vi "NF87XX.ProcCases.vi"(0 "i ref in":refnum<vi>, 1 "selector":string, 2 "Data":T1, 3 "call cluster":T2={"Object"="", "Selector"="", "CallType"=enum."synchronous", "Async Object"="", "Async Selector"="", "Data Descriptor"="", "Data"=[], "Error #"=0, "Expire"=0}, 5 "error in":errorcluster) -> (14 "i ref out":refnum<vi>, 17 "answer cluster":T2={"Object"="", "Selector"="", "CallType"=enum."synchronous", "Async Object"="", "Async Selector"="", "Data Descriptor"="", "Data"=[], "Error #"=0, "Expire"=0}, 19 "error out":errorcluster)   [LabVIEW 2014, in "NF87XX.lvlib"]
doc: "This method is called by a process from within the default case in the event loop. The methods of a class that are linked to events will be called from THIS method. Add your code here."
uses:
  NF87XX.lvlib
  CS_Core/CSSystem/CoreDefs/CoreDefs.call_type.ctl
  CS_Core/BaseProcess/BaseProcess.descriptor string definition.ctl
  CS_Core/CSSystem/CoreDefs/CoreDefs.rawDataType.ctl
  NF87XX.motor Type.ctl
  CS_Core/CSSystem/CoreLib/CoreLib.string 2 byte array.vi
  CS_Core/CSSystem/CoreLib/CoreLib.byte array 2 string.vi
  CS_Core/CSSystem/CoreLib/CoreLib.byte array 2 int.vi
  CS_Core/CSSystem/CoreLib/CoreLib.byte array 2 short.vi
  CS_Core/CSSystem/CoreLib/CoreLib.double 2 byte array.vi
  CS_Core/CSSystem/CoreLib/CoreLib.byte array 2 double.vi
  CS_Core/CSSystem/CoreLib/CoreLib.int 2 byte array.vi
  CS_Core/CSSystem/CoreLib/CoreLib.short array 2 byte array.vi
  CS_Core/CSSystem/CoreLib/CoreLib.short 2 byte array.vi
  CS_Core/BaseProcess/BaseProcess.lvlib
  CS_Core/CSSystem/CoreLib/CoreLib.lvlib
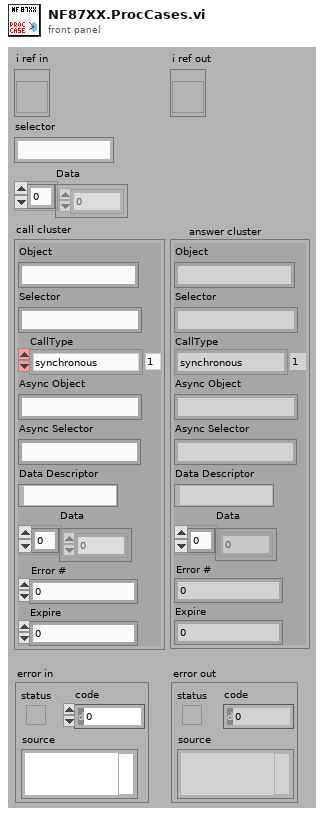
[diagram p1: front panel]
types:
  T1 = typedef "CoreDefs.rawDataType.ctl" = i8[]
  T2 = typedef "CoreDefs.call_type.ctl" = cluster{"Object":string, "Selector":string, "CallType":enum16{"simple", "synchronous", "asynchronous"}, "Async Object":string, "Async Selector":string, "Data Descriptor":T3, "Data":T1, "Error #":i32, "Expire":u32}
  T3 = typedef "BaseProcess.lvlib/BaseProcess.descriptor string definition.ctl" = string
  T4 = typedef "NF87XX.lvlib/NF87XX.motor Type.ctl" = enum16{"Standard Picomotor", "Tiny Picomotor", "not defined"}
  T5 = typedef "NF87XX.lvlib/NF87XX.driver Type.ctl" = enum16{"not defined", "3-ch open loop drv", "1-ch closed loop drv"}
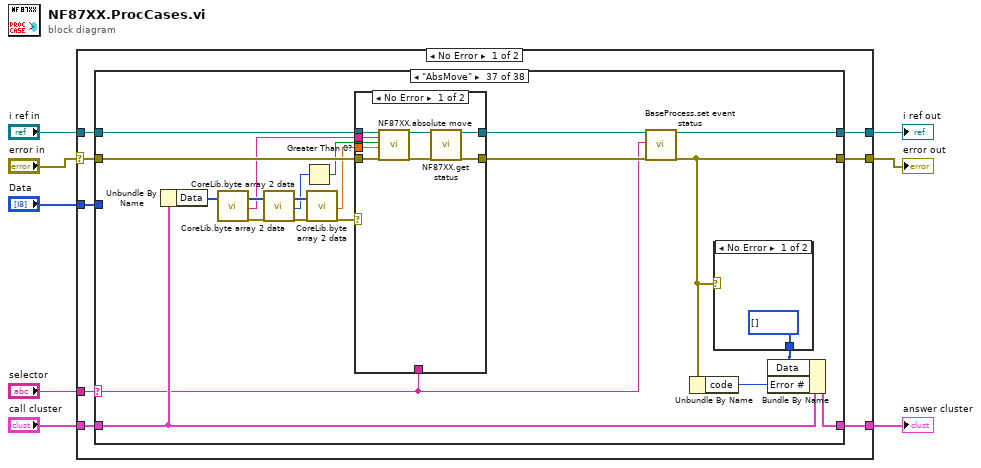
[diagram p0: block diagram]
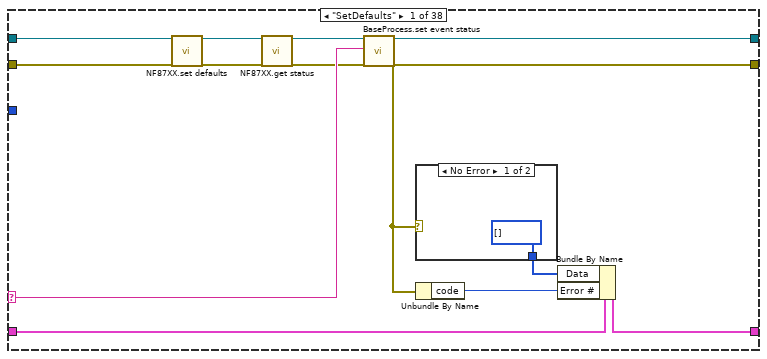
[diagram p2: hidden frame]
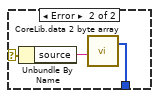
[diagram p3: hidden frame]
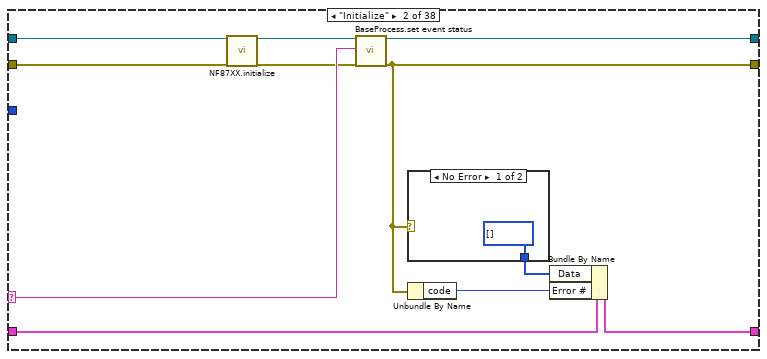
[diagram p4: hidden frame]
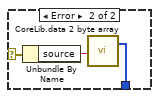
[diagram p5: hidden frame]
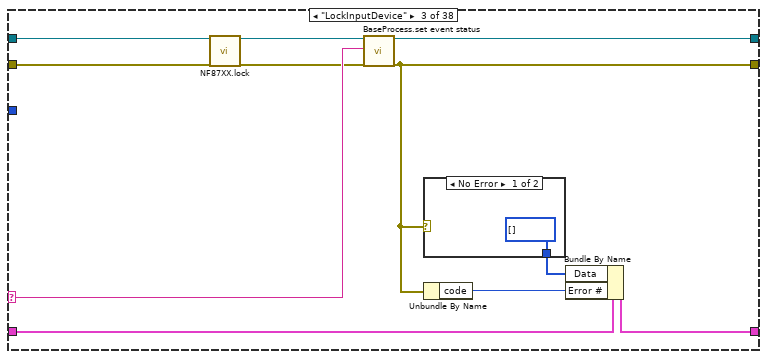
[diagram p6: hidden frame]
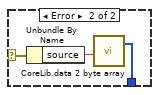
[diagram p7: hidden frame]
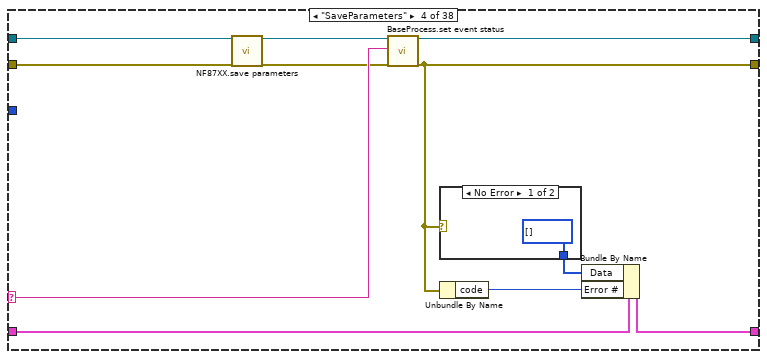
[diagram p8: hidden frame]
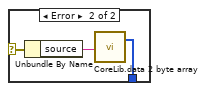
[diagram p9: hidden frame]
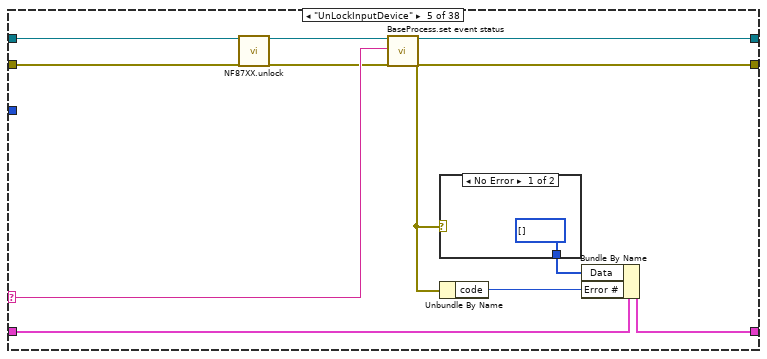
[diagram p10: hidden frame]
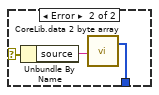
[diagram p11: hidden frame]
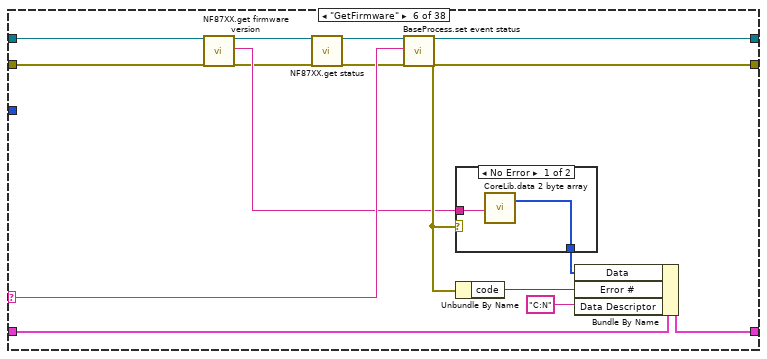
[diagram p12: hidden frame]
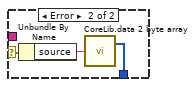
[diagram p13: hidden frame]
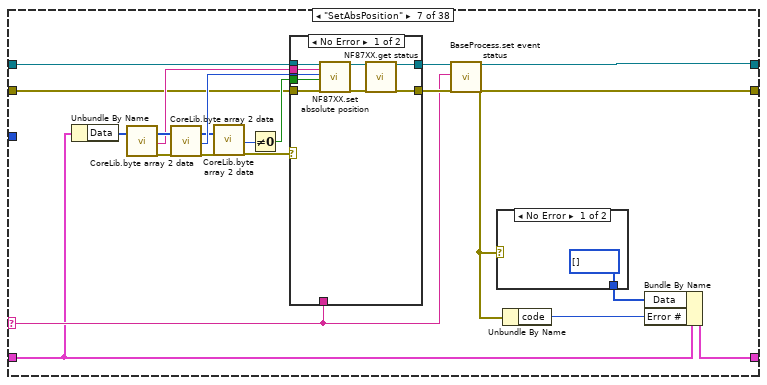
[diagram p14: hidden frame]
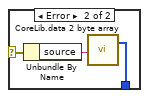
[diagram p15: hidden frame]
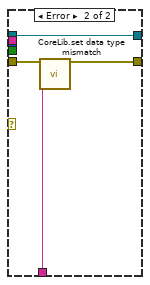
[diagram p16: hidden frame]
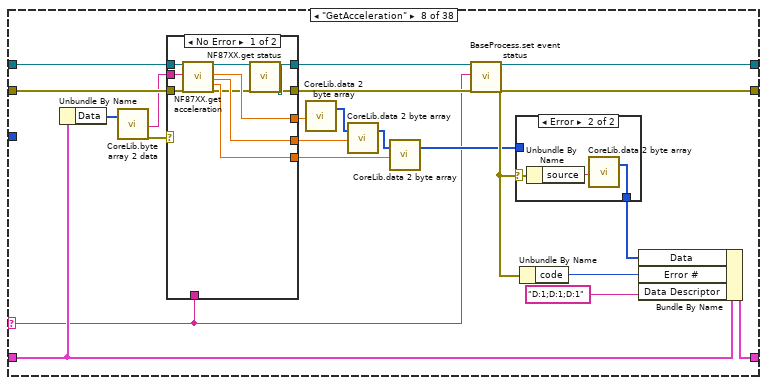
[diagram p17: hidden frame]
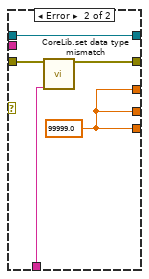
[diagram p18: hidden frame]
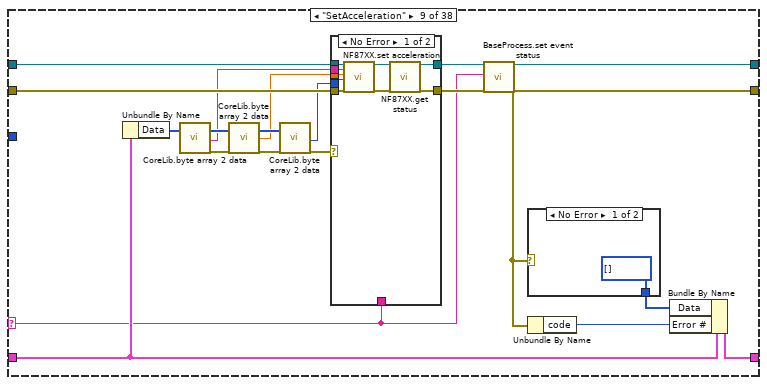
[diagram p20: hidden frame]
diagram:
  n1 = case shown="No Error" "error in" {
    selector: "error in" -> [w10 w1085]
    tunnel: "selector" -> [w16 _]
    tunnel: [w15 w1086] -> w7
    tunnel: "call cluster" -> [w14 w1086]
    tunnel: "i ref in" -> [w13 w1087]
    tunnel: [w12 w1087] -> w4
    tunnel: [w11 w1085] -> w3
    tunnel: "Data" -> [w9 _]
    frame No Error {
      n2 = case shown="\"AbsMove\"" w16 {
        selector: w16 -> [w25 w40 w55 w70 w85 w104 w116 w152 w203 w230 w271 w306 w319 w353 w386 w413 w451 w482 w511 w528 w540 w592 w624 w656 w664 w710 w743 w763 w783 w831 w856 w908 w944 w964 w973 w1001 w1042 w1076]
        tunnel: w13 -> [w23 w38 w53 w68 w83 w101 w120 w168 w211 w241 w279 w303 w331 w365 w388 w422 w459 w490 w518 w535 w556 w599 w631 w652 w674 w717 w741 w756 w795 w838 w872 w915 w942 w962 w975 w1009 w1050 w1074]
        tunnel: [w24 w39 w54 w69 w84 w103 w118 w169 w202 w242 w270 w305 w333 w367 w394 w423 w450 w481 w510 w527 w557 w591 w623 w655 w677 w709 w742 w762 w796 w830 w873 w907 w943 w963 w980 w1000 w1041 w1075] -> w12
        tunnel: w14 -> [w28 w43 w58 w73 w88 w107 w115 w155 w208 w232 w276 w309 w324 w358 w389 w416 w456 w487 w516 w533 w543 w590 w622 w654 w668 w708 w746 w753 w786 w829 w859 w906 w947 w967 w976 w1006 w1047 w1079]
        tunnel: [w27 w42 w57 w72 w87 w106 w114 w171 w207 w244 w275 w308 w326 w360 w396 w425 w455 w486 w515 w532 w559 w596 w628 w658 w679 w714 w745 w765 w798 w835 w875 w912 w946 w966 w977 w1005 w1046 w1078] -> w15
        tunnel: w10 -> [w22 w36 w51 w66 w81 w100 w119 w167 w210 w240 w278 w302 w332 w366 w387 w420 w458 w489 w508 w525 w555 w598 w630 w651 w675 w716 w740 w757 w794 w837 w871 w914 w941 w961 w979 w1008 w1049 w1073]
        tunnel: [w26 w41 w56 w71 w86 w105 w117 w170 w204 w243 w272 w307 w325 w359 w395 w424 w452 w483 w512 w529 w558 w593 w625 w657 w678 w711 w744 w764 w797 w832 w874 w909 w945 w965 w978 w1002 w1043 w1077] -> w11
        tunnel: w9 -> [_ _ _ _ _ _ _ _ _ _ _ _ _ _ _ _ _ _ _ _ _ _ _ _ _ _ _ _ _ _ _ _ _ _ w974 _ _ _]
        frame "SetDefaults" {
          n3 = call "NF87XX.set defaults.vi"("i ref in"=w23, "error in (no error)"=w22) -> ("i ref out"=w20:refnum<vi>, "error out"=w18:errorcluster)  [unwired: 16 in]
          n4 = call "NF87XX.get status.vi"("i ref in"=w20, "error in (no error)"=w18) -> ("i ref out"=w19:refnum<vi>, "error out"=w17:errorcluster)  [unwired: 15 in, 1 out]
          n5 = call "BaseProcess.set event status.vi"("i ref in"=w19, "EventStatus"=w25, "error in (no error)"=w17) -> ("i ref out"=w24:refnum<vi>, "error out"=w26:errorcluster)  [unwired: 14 in, 1 out]
          n6 = case shown="No Error" w26 {
            selector: w26 -> [_ w33]
            tunnel: [T1 [] ("byteArray out") w31] -> w21
            frame No Error {
            }
            frame Error {
              n7 = Unbundle By Name(w33) -> ("source"=w32:string)
              n8 = call-poly "CoreLib.data 2 byte array.vi"("string"=w32) -> ("byteArray out"=w31:T1)  [unwired: 18 in]
            }
          }
          n9 = Unbundle By Name(w26) -> ("code"=w29:i32)
          n10 = Bundle By Name(cluster=w28, "Data"=w21, "Error #"=w29) -> (w27:T2)
        }
        frame "Initialize" {
          n11 = call "NF87XX.initialize.vi"("i ref in"=w38, "error in (no error)"=w36) -> ("i ref out"=w37:refnum<vi>, "error out"=w34:errorcluster)  [unwired: 16 in]
          n12 = call "BaseProcess.set event status.vi"("i ref in"=w37, "EventStatus"=w40, "error in (no error)"=w34) -> ("i ref out"=w39:refnum<vi>, "error out"=w41:errorcluster)  [unwired: 14 in, 1 out]
          n13 = case shown="No Error" w41 {
            selector: w41 -> [_ w48]
            tunnel: [T1 [] ("byteArray out") w46] -> w35
            frame No Error {
            }
            frame Error {
              n14 = Unbundle By Name(w48) -> ("source"=w47:string)
              n15 = call-poly "CoreLib.data 2 byte array.vi"("string"=w47) -> ("byteArray out"=w46:T1)  [unwired: 18 in]
            }
          }
          n16 = Unbundle By Name(w41) -> ("code"=w44:i32)
          n17 = Bundle By Name(cluster=w43, "Data"=w35, "Error #"=w44) -> (w42:T2)
        }
        frame "LockInputDevice" {
          n18 = call "NF87XX.lock.vi"("i ref in"=w53, "error in (no error)"=w51) -> ("i ref out"=w52:refnum<vi>, "error out"=w50:errorcluster)  [unwired: 16 in]
          n19 = call "BaseProcess.set event status.vi"("i ref in"=w52, "EventStatus"=w55, "error in (no error)"=w50) -> ("i ref out"=w54:refnum<vi>, "error out"=w56:errorcluster)  [unwired: 14 in, 1 out]
          n20 = case shown="No Error" w56 {
            selector: w56 -> [_ w63]
            tunnel: [T1 [] ("byteArray out") w61] -> w49
            frame No Error {
            }
            frame Error {
              n21 = Unbundle By Name(w63) -> ("source"=w62:string)
              n22 = call-poly "CoreLib.data 2 byte array.vi"("string"=w62) -> ("byteArray out"=w61:T1)  [unwired: 18 in]
            }
          }
          n23 = Unbundle By Name(w56) -> ("code"=w59:i32)
          n24 = Bundle By Name(cluster=w58, "Data"=w49, "Error #"=w59) -> (w57:T2)
        }
        frame "SaveParameters" {
          n25 = call "NF87XX.save parameters.vi"("i ref in"=w68, "error in (no error)"=w66) -> ("i ref out"=w67:refnum<vi>, "error out"=w65:errorcluster)  [unwired: 16 in]
          n26 = call "BaseProcess.set event status.vi"("i ref in"=w67, "EventStatus"=w70, "error in (no error)"=w65) -> ("i ref out"=w69:refnum<vi>, "error out"=w71:errorcluster)  [unwired: 14 in, 1 out]
          n27 = case shown="No Error" w71 {
            selector: w71 -> [_ w78]
            tunnel: [T1 [] ("byteArray out") w76] -> w64
            frame No Error {
            }
            frame Error {
              n28 = Unbundle By Name(w78) -> ("source"=w77:string)
              n29 = call-poly "CoreLib.data 2 byte array.vi"("string"=w77) -> ("byteArray out"=w76:T1)  [unwired: 18 in]
            }
          }
          n30 = Unbundle By Name(w71) -> ("code"=w74:i32)
          n31 = Bundle By Name(cluster=w73, "Data"=w64, "Error #"=w74) -> (w72:T2)
        }
        frame "UnLockInputDevice" {
          n32 = call "NF87XX.unlock.vi"("i ref in"=w83, "error in (no error)"=w81) -> ("i ref out"=w82:refnum<vi>, "error out"=w80:errorcluster)  [unwired: 16 in]
          n33 = call "BaseProcess.set event status.vi"("i ref in"=w82, "EventStatus"=w85, "error in (no error)"=w80) -> ("i ref out"=w84:refnum<vi>, "error out"=w86:errorcluster)  [unwired: 14 in, 1 out]
          n34 = case shown="No Error" w86 {
            selector: w86 -> [_ w93]
            tunnel: [T1 [] ("byteArray out") w91] -> w79
            frame No Error {
            }
            frame Error {
              n35 = Unbundle By Name(w93) -> ("source"=w92:string)
              n36 = call-poly "CoreLib.data 2 byte array.vi"("string"=w92) -> ("byteArray out"=w91:T1)  [unwired: 18 in]
            }
          }
          n37 = Unbundle By Name(w86) -> ("code"=w89:i32)
          n38 = Bundle By Name(cluster=w88, "Data"=w79, "Error #"=w89) -> (w87:T2)
        }
        frame "GetFirmware" {
          n39 = call "NF87XX.get firmware version.vi"("i ref in"=w101, "error in (no error)"=w100) -> ("i ref out"=w97:refnum<vi>, "firmware version"=w99:string, "error out"=w95:errorcluster)  [unwired: 15 in]
          n40 = call "NF87XX.get status.vi"("i ref in"=w97, "error in (no error)"=w95) -> ("i ref out"=w96:refnum<vi>, "error out"=w94:errorcluster)  [unwired: 15 in, 1 out]
          n41 = call "BaseProcess.set event status.vi"("i ref in"=w96, "EventStatus"=w104, "error in (no error)"=w94) -> ("i ref out"=w103:refnum<vi>, "error out"=w105:errorcluster)  [unwired: 14 in, 1 out]
          n42 = case shown="No Error" w105 {
            selector: w105 -> [_ w113]
            tunnel: w99 -> [w110 _]
            tunnel: [w109 w111] -> w98
            frame No Error {
              n43 = call-poly "CoreLib.data 2 byte array.vi"("string"=w110) -> ("byteArray out"=w109:T1)  [unwired: 18 in]
            }
            frame Error {
              n44 = Unbundle By Name(w113) -> ("source"=w112:string)
              n45 = call-poly "CoreLib.data 2 byte array.vi"("string"=w112) -> ("byteArray out"=w111:T1)  [unwired: 18 in]
            }
          }
          n46 = Unbundle By Name(w105) -> ("code"=w108:i32)
          n47 = Bundle By Name(cluster=w107, "Data"=w98, "Error #"=w108, "Data Descriptor"="C:N") -> (w106:T2)
        }
        frame "SetAbsPosition" {
          n48 = Unbundle By Name(w115) -> ("Data"=w124:T1)
          n49 = call-poly "CoreLib.byte array 2 data.vi"("byteArray"=w124) -> ("byteArray out"=w123:T1, "string"=w121:string, "error out"=w122:errorcluster)  [unwired: 16 in]
          n50 = call-poly "CoreLib.byte array 2 data.vi"("byteArray"=w123, "error in (no error)"=w122) -> ("byteArray out"=w125:T1, "i32"=w126:i32, "error out"=w129:errorcluster)  [unwired: 15 in]
          n51 = call-poly "CoreLib.byte array 2 data.vi"("byteArray"=w125, "error in (no error)"=w129) -> ("i16"=w130:i16, "error out"=w128:errorcluster)  [unwired: 15 in, 1 out]
          n52 = Not Equal To 0?(x=w130) -> (x != 0?=w127:bool)
          n53 = case shown="No Error" w128 {
            tunnel: [w141 w151] -> w133
            tunnel: w120 -> [w146 w151]
            tunnel: w119 -> [w147 w150]
            tunnel: [w139 w149] -> w132
            tunnel: w116 -> [_ w148]
            tunnel: w126 -> [w145 _]
            tunnel: w127 -> [w144 _]
            tunnel: w121 -> [w143 _]
            frame No Error {
              n54 = call "NF87XX.set absolute position.vi"("i ref in"=w146, "System"=w143, "position"=w145, "Go immediately?"=w144, "error in (no error)"=w147) -> ("i ref out"=w142:refnum<vi>, "error out"=w140:errorcluster)  [unwired: 13 in]
              n55 = call "NF87XX.get status.vi"("i ref in"=w142, "error in (no error)"=w140) -> ("i ref out"=w141:refnum<vi>, "error out"=w139:errorcluster)  [unwired: 15 in, 1 out]
            }
            frame Error {
              n56 = call "CoreLib.set data type mismatch.vi"("error in (no error)"=w150, "error source"=w148) -> ("error out"=w149:errorcluster)  [unwired: 17 in]
            }
          }
          n57 = call "BaseProcess.set event status.vi"("i ref in"=w133, "EventStatus"=w116, "error in (no error)"=w132) -> ("i ref out"=w118:refnum<vi>, "error out"=w117:errorcluster)  [unwired: 14 in, 1 out]
          n58 = case shown="No Error" w117 {
            selector: w117 -> [_ w138]
            tunnel: [T1 [] ("byteArray out") w136] -> w131
            frame No Error {
            }
            frame Error {
              n59 = Unbundle By Name(w138) -> ("source"=w137:string)
              n60 = call-poly "CoreLib.data 2 byte array.vi"("string"=w137) -> ("byteArray out"=w136:T1)  [unwired: 18 in]
            }
          }
          n61 = Unbundle By Name(w117) -> ("code"=w134:i32)
          n62 = Bundle By Name(cluster=w115, "Data"=w131, "Error #"=w134) -> (w114:T2)
        }
        frame "GetAcceleration" {
          n63 = Unbundle By Name(w155) -> ("Data"=w156:T1)
          n64 = call-poly "CoreLib.byte array 2 data.vi"("byteArray"=w156) -> ("string"=w154:string, "error out"=w153:errorcluster)  [unwired: 16 in, 1 out]
          n65 = case shown="No Error" w153 {
            tunnel: w168 -> [w182 w185]
            tunnel: w167 -> [w181 w187]
            tunnel: [w173 w186] -> w166
            tunnel: [w175 w185] -> w165
            tunnel: [w180 w183] -> w163
            tunnel: [w179 w183] -> w162
            tunnel: [w178 w183] -> w161
            tunnel: w154 -> [w177 _]
            tunnel: w152 -> [_ w184]
            frame No Error {
              n66 = call "NF87XX.get acceleration.vi"("i ref in"=w182, "System"=w177, "error in (no error)"=w181) -> ("i ref out"=w176:refnum<vi>, "acceleration Mot 0 [steps/s²]"=w180:dbl, "acceleration Mot 1 [steps/s²]"=w179:dbl, "acceleration Mot 2 [steps/s²]"=w178:dbl, "error out"=w174:errorcluster)  [unwired: 12 in]
              n67 = call "NF87XX.get status.vi"("i ref in"=w176, "error in (no error)"=w174) -> ("i ref out"=w175:refnum<vi>, "error out"=w173:errorcluster)  [unwired: 15 in, 1 out]
            }
            frame Error {
              w183 = 99999.0 ("acceleration Mot 0 [steps/s²]")
              n68 = call "CoreLib.set data type mismatch.vi"("error in (no error)"=w187, "error source"=w184) -> ("error out"=w186:errorcluster)  [unwired: 17 in]
            }
          }
          n69 = call-poly "CoreLib.data 2 byte array.vi"("f64"=w163) -> ("byteArray out"=w160:T1)  [unwired: 18 in]
          n70 = call-poly "CoreLib.data 2 byte array.vi"("byteArray"=w160, "f64"=w162) -> ("byteArray out"=w159:T1)  [unwired: 17 in]
          n71 = call-poly "CoreLib.data 2 byte array.vi"("byteArray"=w159, "f64"=w161) -> ("byteArray out"=w158:T1)  [unwired: 17 in]
          n72 = call "BaseProcess.set event status.vi"("i ref in"=w165, "EventStatus"=w152, "error in (no error)"=w166) -> ("i ref out"=w169:refnum<vi>, "error out"=w170:errorcluster)  [unwired: 14 in, 1 out]
          n73 = case shown="Error" w170 {
            selector: w170 -> [_ w191]
            tunnel: w158 -> [w188 _]
            tunnel: [w188 w189] -> w157
            frame No Error {
            }
            frame Error {
              n74 = Unbundle By Name(w191) -> ("source"=w190:string)
              n75 = call-poly "CoreLib.data 2 byte array.vi"("string"=w190) -> ("byteArray out"=w189:T1)  [unwired: 18 in]
            }
          }
          n76 = Unbundle By Name(w170) -> ("code"=w172:i32)
          n77 = Bundle By Name(cluster=w155, "Data"=w157, "Error #"=w172, "Data Descriptor"="D:1;D:1;D:1") -> (w171:T2)
        }
        frame "SetAcceleration" {
          n78 = Unbundle By Name(w208) -> ("Data"=w193:T1)
          n79 = call-poly "CoreLib.byte array 2 data.vi"("byteArray"=w193) -> ("byteArray out"=w194:T1, "string"=w192:string, "error out"=w195:errorcluster)  [unwired: 16 in]
          n80 = call-poly "CoreLib.byte array 2 data.vi"("byteArray"=w194, "error in (no error)"=w195) -> ("byteArray out"=w201:T1, "d64"=w198:dbl, "error out"=w200:errorcluster)  [unwired: 15 in]
          n81 = call-poly "CoreLib.byte array 2 data.vi"("byteArray"=w201, "error in (no error)"=w200) -> ("i32"=w197:i32, "error out"=w199:errorcluster)  [unwired: 15 in, 1 out]
          n82 = case shown="No Error" w199 {
            tunnel: [w218 w228] -> w206
            tunnel: w211 -> [w224 w228]
            tunnel: w210 -> [w223 w227]
            tunnel: [w216 w226] -> w205
            tunnel: w203 -> [_ w225]
            tunnel: w198 -> [w222 _]
            tunnel: w197 -> [w221 _]
            tunnel: w192 -> [w220 _]
            frame No Error {
              n83 = call "NF87XX.set acceleration.vi"("i ref in"=w224, "System"=w220, "acceleration (16 .. 20000)"=w222, "Motor (0,1,2)"=w221, "error in (no error)"=w223) -> ("i ref out"=w219:refnum<vi>, "error out"=w217:errorcluster)  [unwired: 13 in]
              n84 = call "NF87XX.get status.vi"("i ref in"=w219, "error in (no error)"=w217) -> ("i ref out"=w218:refnum<vi>, "error out"=w216:errorcluster)  [unwired: 15 in, 1 out]
            }
            frame Error {
              n85 = call "CoreLib.set data type mismatch.vi"("error in (no error)"=w227, "error source"=w225) -> ("error out"=w226:errorcluster)  [unwired: 17 in]
            }
          }
          n86 = call "BaseProcess.set event status.vi"("i ref in"=w206, "EventStatus"=w203, "error in (no error)"=w205) -> ("i ref out"=w202:refnum<vi>, "error out"=w204:errorcluster)  [unwired: 14 in, 1 out]
          n87 = case shown="No Error" w204 {
            selector: w204 -> [_ w215]
            tunnel: [T1 [] ("byteArray out") w213] -> w196
            frame No Error {
            }
            frame Error {
              n88 = Unbundle By Name(w215) -> ("source"=w214:string)
              n89 = call-poly "CoreLib.data 2 byte array.vi"("string"=w214) -> ("byteArray out"=w213:T1)  [unwired: 18 in]
            }
          }
          n90 = Unbundle By Name(w204) -> ("code"=w209:i32)
          n91 = Bundle By Name(cluster=w208, "Data"=w196, "Error #"=w209) -> (w207:T2)
        }
        frame "GetChannel" {
          n92 = Unbundle By Name(w232) -> ("Data"=w233:T1)
          n93 = call-poly "CoreLib.byte array 2 data.vi"("byteArray"=w233) -> ("string"=w229:string, "error out"=w231:errorcluster)  [unwired: 16 in, 1 out]
          n94 = case shown="No Error" w231 {
            tunnel: w241 -> [w253 w256]
            tunnel: w240 -> [w252 w258]
            tunnel: [w248 w257] -> w239
            tunnel: [w246 w256] -> w238
            tunnel: [w251 99999 ("Channel")] -> w234
            tunnel: w230 -> [_ w255]
            tunnel: w229 -> [w250 _]
            frame No Error {
              n95 = call "NF87XX.get channel.vi"("i ref in"=w253, "System"=w250, "error in (no error)"=w252) -> ("i ref out"=w247:refnum<vi>, "Channel"=w251:i32, "error out"=w249:errorcluster)  [unwired: 14 in]
              n96 = call "NF87XX.get status.vi"("i ref in"=w247, "error in (no error)"=w249) -> ("i ref out"=w246:refnum<vi>, "error out"=w248:errorcluster)  [unwired: 15 in, 1 out]
            }
            frame Error {
              n97 = call "CoreLib.set data type mismatch.vi"("error in (no error)"=w258, "error source"=w255) -> ("error out"=w257:errorcluster)  [unwired: 17 in]
            }
          }
          n98 = call-poly "CoreLib.data 2 byte array.vi"("i32"=w234) -> ("byteArray out"=w236:T1)  [unwired: 18 in]
          n99 = call "BaseProcess.set event status.vi"("i ref in"=w238, "EventStatus"=w230, "error in (no error)"=w239) -> ("i ref out"=w242:refnum<vi>, "error out"=w243:errorcluster)  [unwired: 14 in, 1 out]
          n100 = case shown="Error" w243 {
            selector: w243 -> [_ w262]
            tunnel: w236 -> [w259 _]
            tunnel: [w259 w260] -> w235
            frame No Error {
            }
            frame Error {
              n101 = Unbundle By Name(w262) -> ("source"=w261:string)
              n102 = call-poly "CoreLib.data 2 byte array.vi"("string"=w261) -> ("byteArray out"=w260:T1)  [unwired: 18 in]
            }
          }
          n103 = Unbundle By Name(w243) -> ("code"=w245:i32)
          n104 = Bundle By Name(cluster=w232, "Data"=w235, "Error #"=w245, "Data Descriptor"="I:1") -> (w244:T2)
        }
        frame "SetChannel" {
          n105 = Unbundle By Name(w276) -> ("Data"=w266:T1)
          n106 = call-poly "CoreLib.byte array 2 data.vi"("byteArray"=w266) -> ("byteArray out"=w265:T1, "string"=w263:string, "error out"=w264:errorcluster)  [unwired: 16 in]
          n107 = call-poly "CoreLib.byte array 2 data.vi"("byteArray"=w265, "error in (no error)"=w264) -> ("i32"=w268:i32, "error out"=w269:errorcluster)  [unwired: 15 in, 1 out]
          n108 = case shown="No Error" w269 {
            tunnel: [w286 w295] -> w274
            tunnel: w279 -> [w291 w295]
            tunnel: w278 -> [w290 w294]
            tunnel: [w284 w293] -> w273
            tunnel: w271 -> [_ w292]
            tunnel: w268 -> [w289 _]
            tunnel: w263 -> [w288 _]
            frame No Error {
              n109 = call "NF87XX.set axis channel.vi"("i ref in"=w291, "System"=w288, "channel"=w289, "error in (no error)"=w290) -> ("i ref out"=w287:refnum<vi>, "error out"=w285:errorcluster)  [unwired: 14 in]
              n110 = call "NF87XX.get status.vi"("i ref in"=w287, "error in (no error)"=w285) -> ("i ref out"=w286:refnum<vi>, "error out"=w284:errorcluster)  [unwired: 15 in, 1 out]
            }
            frame Error {
              n111 = call "CoreLib.set data type mismatch.vi"("error in (no error)"=w294, "error source"=w292) -> ("error out"=w293:errorcluster)  [unwired: 17 in]
            }
          }
          n112 = call "BaseProcess.set event status.vi"("i ref in"=w274, "EventStatus"=w271, "error in (no error)"=w273) -> ("i ref out"=w270:refnum<vi>, "error out"=w272:errorcluster)  [unwired: 14 in, 1 out]
          n113 = case shown="No Error" w272 {
            selector: w272 -> [_ w283]
            tunnel: [T1 [] ("byteArray out") w281] -> w267
            frame No Error {
            }
            frame Error {
              n114 = Unbundle By Name(w283) -> ("source"=w282:string)
              n115 = call-poly "CoreLib.data 2 byte array.vi"("string"=w282) -> ("byteArray out"=w281:T1)  [unwired: 18 in]
            }
          }
          n116 = Unbundle By Name(w272) -> ("code"=w277:i32)
          n117 = Bundle By Name(cluster=w276, "Data"=w267, "Error #"=w277) -> (w275:T2)
        }
        frame "GetDriverType" {
          n118 = call "NF87XX.get driver type.vi"("i ref in"=w303, "error in (no error)"=w302) -> ("i ref out"=w297:refnum<vi>, "Driver Types"=w300:T5[], "error out"=w299:errorcluster)  [unwired: 15 in]
          n119 = call "NF87XX.get status.vi"("i ref in"=w297, "error in (no error)"=w299) -> ("i ref out"=w296:refnum<vi>, "error out"=w298:errorcluster)  [unwired: 15 in, 1 out]
          n120 = call "BaseProcess.set event status.vi"("i ref in"=w296, "EventStatus"=w306, "error in (no error)"=w298) -> ("i ref out"=w305:refnum<vi>, "error out"=w307:errorcluster)  [unwired: 14 in, 1 out]
          n121 = case shown="No Error" w307 {
            selector: w307 -> [_ w315]
            tunnel: [w312 w313] -> w301
            tunnel: w300 -> [w311 _]
            frame No Error {
              n122 = call-poly "CoreLib.data 2 byte array.vi"("byteArray"=w311) -> ("byteArray out"=w312:T1)  [unwired: 18 in]
            }
            frame Error {
              n123 = Unbundle By Name(w315) -> ("source"=w314:string)
              n124 = call-poly "CoreLib.data 2 byte array.vi"("string"=w314) -> ("byteArray out"=w313:T1)  [unwired: 18 in]
            }
          }
          n125 = Unbundle By Name(w307) -> ("code"=w310:i32)
          n126 = Bundle By Name(cluster=w309, "Data"=w301, "Error #"=w310, "Data Descriptor"="S:N") -> (w308:T2)
        }
        frame "FindIndexMark" {
          n127 = Unbundle By Name(w324) -> ("Data"=w323:T1)
          n128 = call-poly "CoreLib.byte array 2 data.vi"("byteArray"=w323) -> ("byteArray out"=w322:T1, "string"=w317:string, "error out"=w316:errorcluster)  [unwired: 16 in]
          n129 = call-poly "CoreLib.byte array 2 data.vi"("byteArray"=w322, "error in (no error)"=w316) -> ("i16"=w320:i16, "error out"=w321:errorcluster)  [unwired: 15 in, 1 out]
          n130 = Not Equal To 0?(x=w320) -> (x != 0?=w318:bool)
          n131 = case shown="No Error" w321 {
            tunnel: w332 -> [w341 w344]
            tunnel: w331 -> [w340 w345]
            tunnel: [w334 w345] -> w330
            tunnel: [w336 w343] -> w329
            tunnel: w319 -> [_ w342]
            tunnel: w318 -> [w339 _]
            tunnel: w317 -> [w338 _]
            frame No Error {
              n132 = call "NF87XX.Drive to Indexmark.vi"("i ref in"=w340, "System"=w338, "Forward?"=w339, "error in (no error)"=w341) -> ("i ref out"=w335:refnum<vi>, "error out"=w337:errorcluster)  [unwired: 14 in]
              n133 = call "NF87XX.get status.vi"("i ref in"=w335, "error in (no error)"=w337) -> ("i ref out"=w334:refnum<vi>, "error out"=w336:errorcluster)  [unwired: 15 in, 1 out]
            }
            frame Error {
              n134 = call "CoreLib.set data type mismatch.vi"("error in (no error)"=w344, "error source"=w342) -> ("error out"=w343:errorcluster)  [unwired: 17 in]
            }
          }
          n135 = call "BaseProcess.set event status.vi"("i ref in"=w330, "EventStatus"=w319, "error in (no error)"=w329) -> ("i ref out"=w333:refnum<vi>, "error out"=w325:errorcluster)  [unwired: 14 in, 1 out]
          n136 = case shown="No Error" w325 {
            selector: w325 -> [_ w349]
            tunnel: [T1 [] ("byteArray out") w347] -> w327
            frame No Error {
            }
            frame Error {
              n137 = Unbundle By Name(w349) -> ("source"=w348:string)
              n138 = call-poly "CoreLib.data 2 byte array.vi"("string"=w348) -> ("byteArray out"=w347:T1)  [unwired: 18 in]
            }
          }
          n139 = Unbundle By Name(w325) -> ("code"=w328:i32)
          n140 = Bundle By Name(cluster=w324, "Data"=w327, "Error #"=w328) -> (w326:T2)
        }
        frame "FindLimit" {
          n141 = Unbundle By Name(w358) -> ("Data"=w357:T1)
          n142 = call-poly "CoreLib.byte array 2 data.vi"("byteArray"=w357) -> ("byteArray out"=w356:T1, "string"=w351:string, "error out"=w350:errorcluster)  [unwired: 16 in]
          n143 = call-poly "CoreLib.byte array 2 data.vi"("byteArray"=w356, "error in (no error)"=w350) -> ("i16"=w354:i16, "error out"=w355:errorcluster)  [unwired: 15 in, 1 out]
          n144 = Not Equal To 0?(x=w354) -> (x != 0?=w352:bool)
          n145 = case shown="No Error" w355 {
            tunnel: w366 -> [w375 w378]
            tunnel: w365 -> [w374 w379]
            tunnel: [w370 w379] -> w364
            tunnel: [w368 w377] -> w363
            tunnel: w353 -> [_ w376]
            tunnel: w352 -> [w373 _]
            tunnel: w351 -> [w372 _]
            frame No Error {
              n146 = call "NF87XX.Drive to Limit.vi"("i ref in"=w374, "System"=w372, "Forward?"=w373, "error in (no error)"=w375) -> ("i ref out"=w371:refnum<vi>, "error out"=w369:errorcluster)  [unwired: 14 in]
              n147 = call "NF87XX.get status.vi"("i ref in"=w371, "error in (no error)"=w369) -> ("i ref out"=w370:refnum<vi>, "error out"=w368:errorcluster)  [unwired: 15 in, 1 out]
            }
            frame Error {
              n148 = call "CoreLib.set data type mismatch.vi"("error in (no error)"=w378, "error source"=w376) -> ("error out"=w377:errorcluster)  [unwired: 17 in]
            }
          }
          n149 = call "BaseProcess.set event status.vi"("i ref in"=w364, "EventStatus"=w353, "error in (no error)"=w363) -> ("i ref out"=w367:refnum<vi>, "error out"=w359:errorcluster)  [unwired: 14 in, 1 out]
          n150 = case shown="No Error" w359 {
            selector: w359 -> [_ w383]
            tunnel: [T1 [] ("byteArray out") w381] -> w361
            frame No Error {
            }
            frame Error {
              n151 = Unbundle By Name(w383) -> ("source"=w382:string)
              n152 = call-poly "CoreLib.data 2 byte array.vi"("string"=w382) -> ("byteArray out"=w381:T1)  [unwired: 18 in]
            }
          }
          n153 = Unbundle By Name(w359) -> ("code"=w362:i32)
          n154 = Bundle By Name(cluster=w358, "Data"=w361, "Error #"=w362) -> (w360:T2)
        }
        frame "Start" {
          n155 = Unbundle By Name(w389) -> ("Data"=w392:T1)
          n156 = call-poly "CoreLib.byte array 2 data.vi"("byteArray"=w392) -> ("string"=w391:string, "error out"=w390:errorcluster)  [unwired: 16 in, 1 out]
          n157 = case shown="No Error" w390 {
            tunnel: w388 -> [w404 w406]
            tunnel: w387 -> [w403 w408]
            tunnel: [w398 w407] -> w384
            tunnel: [w400 w406] -> w385
            tunnel: w391 -> [w402 _]
            tunnel: w386 -> [_ w405]
            frame No Error {
              n158 = call "NF87XX.start motion.vi"("i ref in"=w404, "System"=w402, "error in (no error)"=w403) -> ("i ref out"=w401:refnum<vi>, "error out"=w399:errorcluster)  [unwired: 15 in]
              n159 = call "NF87XX.get status.vi"("i ref in"=w401, "error in (no error)"=w399) -> ("i ref out"=w400:refnum<vi>, "error out"=w398:errorcluster)  [unwired: 15 in, 1 out]
            }
            frame Error {
              n160 = call "CoreLib.set data type mismatch.vi"("error in (no error)"=w408, "error source"=w405) -> ("error out"=w407:errorcluster)  [unwired: 17 in]
            }
          }
          n161 = call "BaseProcess.set event status.vi"("i ref in"=w385, "EventStatus"=w386, "error in (no error)"=w384) -> ("i ref out"=w394:refnum<vi>, "error out"=w395:errorcluster)  [unwired: 14 in, 1 out]
          n162 = case shown="Error" w395 {
            selector: w395 -> [_ w412]
            tunnel: [T1 [] ("byteArray out") w410] -> w393
            frame No Error {
            }
            frame Error {
              n163 = Unbundle By Name(w412) -> ("source"=w411:string)
              n164 = call-poly "CoreLib.data 2 byte array.vi"("string"=w411) -> ("byteArray out"=w410:T1)  [unwired: 18 in]
            }
          }
          n165 = Unbundle By Name(w395) -> ("code"=w397:i32)
          n166 = Bundle By Name(cluster=w389, "Data"=w393, "Error #"=w397) -> (w396:T2)
        }
        frame "Halt" {
          n167 = Unbundle By Name(w416) -> ("Data"=w417:T1)
          n168 = call-poly "CoreLib.byte array 2 data.vi"("byteArray"=w417) -> ("string"=w415:string, "error out"=w414:errorcluster)  [unwired: 16 in, 1 out]
          n169 = case shown="No Error" w414 {
            tunnel: w422 -> [w433 w437]
            tunnel: [w427 w437] -> w421
            tunnel: w420 -> [w432 w436]
            tunnel: [w429 w435] -> w419
            tunnel: w415 -> [w431 _]
            tunnel: w413 -> [_ w434]
            frame No Error {
              n170 = call "NF87XX.halt.vi"("i ref in"=w433, "System"=w431, "error in (no error)"=w432) -> ("i ref out"=w428:refnum<vi>, "error out"=w430:errorcluster)  [unwired: 15 in]
              n171 = call "NF87XX.get status.vi"("i ref in"=w428, "error in (no error)"=w430) -> ("i ref out"=w427:refnum<vi>, "error out"=w429:errorcluster)  [unwired: 15 in, 1 out]
            }
            frame Error {
              n172 = call "CoreLib.set data type mismatch.vi"("error in (no error)"=w436, "error source"=w434) -> ("error out"=w435:errorcluster)  [unwired: 17 in]
            }
          }
          n173 = call "BaseProcess.set event status.vi"("i ref in"=w421, "EventStatus"=w413, "error in (no error)"=w419) -> ("i ref out"=w423:refnum<vi>, "error out"=w424:errorcluster)  [unwired: 14 in, 1 out]
          n174 = case shown="No Error" w424 {
            selector: w424 -> [_ w441]
            tunnel: [T1 [] ("byteArray out") w439] -> w418
            frame No Error {
            }
            frame Error {
              n175 = Unbundle By Name(w441) -> ("source"=w440:string)
              n176 = call-poly "CoreLib.data 2 byte array.vi"("string"=w440) -> ("byteArray out"=w439:T1)  [unwired: 18 in]
            }
          }
          n177 = Unbundle By Name(w424) -> ("code"=w426:i32)
          n178 = Bundle By Name(cluster=w416, "Data"=w418, "Error #"=w426) -> (w425:T2)
        }
        frame "EnableDriver" {
          n179 = Unbundle By Name(w456) -> ("Data"=w445:T1)
          n180 = call-poly "CoreLib.byte array 2 data.vi"("byteArray"=w445) -> ("byteArray out"=w444:T1, "string"=w442:string, "error out"=w443:errorcluster)  [unwired: 16 in]
          n181 = call-poly "CoreLib.byte array 2 data.vi"("byteArray"=w444, "error in (no error)"=w443) -> ("i16"=w449:i16, "error out"=w447:errorcluster)  [unwired: 15 in, 1 out]
          n182 = Not Equal To 0?(x=w449) -> (x != 0?=w448:bool)
          n183 = case shown="No Error" w447 {
            tunnel: [w466 w475] -> w454
            tunnel: w459 -> [w471 w475]
            tunnel: w458 -> [w470 w474]
            tunnel: [w464 w473] -> w453
            tunnel: w451 -> [_ w472]
            tunnel: w448 -> [w469 _]
            tunnel: w442 -> [w468 _]
            frame No Error {
              n184 = call "NF87XX.enable driver.vi"("i ref in"=w471, "System"=w468, "Enable Driver"=w469, "error in (no error)"=w470) -> ("i ref out"=w467:refnum<vi>, "error out"=w465:errorcluster)  [unwired: 14 in]
              n185 = call "NF87XX.get status.vi"("i ref in"=w467, "error in (no error)"=w465) -> ("i ref out"=w466:refnum<vi>, "error out"=w464:errorcluster)  [unwired: 15 in, 1 out]
            }
            frame Error {
              n186 = call "CoreLib.set data type mismatch.vi"("error in (no error)"=w474, "error source"=w472) -> ("error out"=w473:errorcluster)  [unwired: 17 in]
            }
          }
          n187 = call "BaseProcess.set event status.vi"("i ref in"=w454, "EventStatus"=w451, "error in (no error)"=w453) -> ("i ref out"=w450:refnum<vi>, "error out"=w452:errorcluster)  [unwired: 14 in, 1 out]
          n188 = case shown="Error" w452 {
            selector: w452 -> [_ w463]
            tunnel: [T1 [] ("byteArray out") w461] -> w446
            frame No Error {
            }
            frame Error {
              n189 = Unbundle By Name(w463) -> ("source"=w462:string)
              n190 = call-poly "CoreLib.data 2 byte array.vi"("string"=w462) -> ("byteArray out"=w461:T1)  [unwired: 18 in]
            }
          }
          n191 = Unbundle By Name(w452) -> ("code"=w457:i32)
          n192 = Bundle By Name(cluster=w456, "Data"=w446, "Error #"=w457) -> (w455:T2)
        }
        frame "EnableJoystick" {
          n193 = Unbundle By Name(w487) -> ("Data"=w477:T1)
          n194 = call-poly "CoreLib.byte array 2 data.vi"("byteArray"=w477) -> ("i16"=w480:i16, "error out"=w478:errorcluster)  [unwired: 16 in, 1 out]
          n195 = Not Equal To 0?(x=w480) -> (x != 0?=w479:bool)
          n196 = case shown="No Error" w478 {
            tunnel: [w497 w505] -> w485
            tunnel: w490 -> [w501 w505]
            tunnel: w489 -> [w500 w504]
            tunnel: [w495 w503] -> w484
            tunnel: w482 -> [_ w502]
            tunnel: w479 -> [w499 _]
            frame No Error {
              n197 = call "NF87XX.enable joystick.vi"("i ref in"=w501, "Enable Joystick"=w499, "error in (no error)"=w500) -> ("i ref out"=w498:refnum<vi>, "error out"=w496:errorcluster)  [unwired: 15 in]
              n198 = call "NF87XX.get status.vi"("i ref in"=w498, "error in (no error)"=w496) -> ("i ref out"=w497:refnum<vi>, "error out"=w495:errorcluster)  [unwired: 15 in, 1 out]
            }
            frame Error {
              n199 = call "CoreLib.set data type mismatch.vi"("error in (no error)"=w504, "error source"=w502) -> ("error out"=w503:errorcluster)  [unwired: 17 in]
            }
          }
          n200 = call "BaseProcess.set event status.vi"("i ref in"=w485, "EventStatus"=w482, "error in (no error)"=w484) -> ("i ref out"=w481:refnum<vi>, "error out"=w483:errorcluster)  [unwired: 14 in, 1 out]
          n201 = case shown="Error" w483 {
            selector: w483 -> [_ w494]
            tunnel: [T1 [] ("byteArray out") w492] -> w476
            frame No Error {
            }
            frame Error {
              n202 = Unbundle By Name(w494) -> ("source"=w493:string)
              n203 = call-poly "CoreLib.data 2 byte array.vi"("string"=w493) -> ("byteArray out"=w492:T1)  [unwired: 18 in]
            }
          }
          n204 = Unbundle By Name(w483) -> ("code"=w488:i32)
          n205 = Bundle By Name(cluster=w487, "Data"=w476, "Error #"=w488) -> (w486:T2)
        }
        frame "SetFineSpeed" {
          n206 = call "NF87XX.set fine speed.vi"("i ref in"=w518, "error in (no error)"=w508) -> ("i ref out"=w507:refnum<vi>, "error out"=w506:errorcluster)  [unwired: 16 in]
          n207 = call "NF87XX.get status.vi"("i ref in"=w507, "error in (no error)"=w506) -> ("i ref out"=w514:refnum<vi>, "error out"=w513:errorcluster)  [unwired: 15 in, 1 out]
          n208 = call "BaseProcess.set event status.vi"("i ref in"=w514, "EventStatus"=w511, "error in (no error)"=w513) -> ("i ref out"=w510:refnum<vi>, "error out"=w512:errorcluster)  [unwired: 14 in, 1 out]
          n209 = case shown="Error" w512 {
            selector: w512 -> [_ w522]
            tunnel: [T1 [] ("byteArray out") w520] -> w509
            frame No Error {
            }
            frame Error {
              n210 = Unbundle By Name(w522) -> ("source"=w521:string)
              n211 = call-poly "CoreLib.data 2 byte array.vi"("string"=w521) -> ("byteArray out"=w520:T1)  [unwired: 18 in]
            }
          }
          n212 = Unbundle By Name(w512) -> ("code"=w517:i32)
          n213 = Bundle By Name(cluster=w516, "Data"=w509, "Error #"=w517) -> (w515:T2)
        }
        frame "SetCoarseSpeed" {
          n214 = call "NF87XX.set coarse speed.vi"("i ref in"=w535, "error in (no error)"=w525) -> ("i ref out"=w524:refnum<vi>, "error out"=w523:errorcluster)  [unwired: 16 in]
          n215 = call "NF87XX.get status.vi"("i ref in"=w524, "error in (no error)"=w523) -> ("i ref out"=w531:refnum<vi>, "error out"=w530:errorcluster)  [unwired: 15 in, 1 out]
          n216 = call "BaseProcess.set event status.vi"("i ref in"=w531, "EventStatus"=w528, "error in (no error)"=w530) -> ("i ref out"=w527:refnum<vi>, "error out"=w529:errorcluster)  [unwired: 14 in, 1 out]
          n217 = case shown="Error" w529 {
            selector: w529 -> [_ w539]
            tunnel: [T1 [] ("byteArray out") w537] -> w526
            frame No Error {
            }
            frame Error {
              n218 = Unbundle By Name(w539) -> ("source"=w538:string)
              n219 = call-poly "CoreLib.data 2 byte array.vi"("string"=w538) -> ("byteArray out"=w537:T1)  [unwired: 18 in]
            }
          }
          n220 = Unbundle By Name(w529) -> ("code"=w534:i32)
          n221 = Bundle By Name(cluster=w533, "Data"=w526, "Error #"=w534) -> (w532:T2)
        }
        frame "GetStartVelocity" {
          n222 = Unbundle By Name(w543) -> ("Data"=w544:T1)
          n223 = call-poly "CoreLib.byte array 2 data.vi"("byteArray"=w544) -> ("string"=w541:string, "error out"=w542:errorcluster)  [unwired: 16 in, 1 out]
          n224 = case shown="No Error" w542 {
            tunnel: w556 -> [w570 w575]
            tunnel: w555 -> [w569 w574]
            tunnel: [w561 w573] -> w554
            tunnel: [w563 w575] -> w553
            tunnel: [w568 w571] -> w548
            tunnel: [w567 w571] -> w547
            tunnel: [w566 w571] -> w546
            tunnel: w541 -> [w565 _]
            tunnel: w540 -> [_ w572]
            frame No Error {
              n225 = call "NF87XX.get start velocity.vi"("i ref in"=w570, "System"=w565, "error in (no error)"=w569) -> ("i ref out"=w564:refnum<vi>, "start velocity Mot 0 [Steps/s]"=w568:dbl, "start velocity Mot 1 [Steps/s]"=w567:dbl, "start velocity Mot 2 [Steps/s]"=w566:dbl, "error out"=w562:errorcluster)  [unwired: 12 in]
              n226 = call "NF87XX.get status.vi"("i ref in"=w564, "error in (no error)"=w562) -> ("i ref out"=w563:refnum<vi>, "error out"=w561:errorcluster)  [unwired: 15 in, 1 out]
            }
            frame Error {
              w571 = 99999.0 ("start velocity Mot 0 [Steps/s]")
              n227 = call "CoreLib.set data type mismatch.vi"("error in (no error)"=w574, "error source"=w572) -> ("error out"=w573:errorcluster)  [unwired: 17 in]
            }
          }
          n228 = call-poly "CoreLib.data 2 byte array.vi"("f64"=w548) -> ("byteArray out"=w551:T1)  [unwired: 18 in]
          n229 = call-poly "CoreLib.data 2 byte array.vi"("byteArray"=w551, "f64"=w547) -> ("byteArray out"=w550:T1)  [unwired: 17 in]
          n230 = call-poly "CoreLib.data 2 byte array.vi"("byteArray"=w550, "f64"=w546) -> ("byteArray out"=w549:T1)  [unwired: 17 in]
          n231 = call "BaseProcess.set event status.vi"("i ref in"=w553, "EventStatus"=w540, "error in (no error)"=w554) -> ("i ref out"=w557:refnum<vi>, "error out"=w558:errorcluster)  [unwired: 14 in, 1 out]
          n232 = case shown="No Error" w558 {
            selector: w558 -> [_ w579]
            tunnel: w549 -> [w576 _]
            tunnel: [w576 w577] -> w545
            frame No Error {
            }
            frame Error {
              n233 = Unbundle By Name(w579) -> ("source"=w578:string)
              n234 = call-poly "CoreLib.data 2 byte array.vi"("string"=w578) -> ("byteArray out"=w577:T1)  [unwired: 18 in]
            }
          }
          n235 = Unbundle By Name(w558) -> ("code"=w560:i32)
          n236 = Bundle By Name(cluster=w543, "Data"=w545, "Error #"=w560, "Data Descriptor"="D:1;D:1;D:1") -> (w559:T2)
        }
        frame "SetStartVelocity" {
          n237 = Unbundle By Name(w590) -> ("Data"=w583:T1)
          n238 = call-poly "CoreLib.byte array 2 data.vi"("byteArray"=w583) -> ("byteArray out"=w582:T1, "string"=w580:string, "error out"=w581:errorcluster)  [unwired: 16 in]
          n239 = call-poly "CoreLib.byte array 2 data.vi"("byteArray"=w582, "error in (no error)"=w581) -> ("byteArray out"=w589:T1, "d64"=w587:dbl, "error out"=w588:errorcluster)  [unwired: 15 in]
          n240 = call-poly "CoreLib.byte array 2 data.vi"("byteArray"=w589, "error in (no error)"=w588) -> ("i32"=w586:i32, "error out"=w585:errorcluster)  [unwired: 15 in, 1 out]
          n241 = case shown="No Error" w585 {
            tunnel: [w606 w616] -> w595
            tunnel: w599 -> [w612 w616]
            tunnel: w598 -> [w611 w615]
            tunnel: [w604 w614] -> w594
            tunnel: w592 -> [_ w613]
            tunnel: w587 -> [w610 _]
            tunnel: w586 -> [w609 _]
            tunnel: w580 -> [w608 _]
            frame No Error {
              n242 = call "NF87XX.set start velocity.vi"("i ref in"=w612, "System"=w608, "start velocity (0 .. 1999)"=w610, "Motor (0,1,2)"=w609, "error in (no error)"=w611) -> ("i ref out"=w607:refnum<vi>, "error out"=w605:errorcluster)  [unwired: 13 in]
              n243 = call "NF87XX.get status.vi"("i ref in"=w607, "error in (no error)"=w605) -> ("i ref out"=w606:refnum<vi>, "error out"=w604:errorcluster)  [unwired: 15 in, 1 out]
            }
            frame Error {
              n244 = call "CoreLib.set data type mismatch.vi"("error in (no error)"=w615, "error source"=w613) -> ("error out"=w614:errorcluster)  [unwired: 17 in]
            }
          }
          n245 = call "BaseProcess.set event status.vi"("i ref in"=w595, "EventStatus"=w592, "error in (no error)"=w594) -> ("i ref out"=w591:refnum<vi>, "error out"=w593:errorcluster)  [unwired: 14 in, 1 out]
          n246 = case shown="No Error" w593 {
            selector: w593 -> [_ w603]
            tunnel: [T1 [] ("byteArray out") w601] -> w584
            frame No Error {
            }
            frame Error {
              n247 = Unbundle By Name(w603) -> ("source"=w602:string)
              n248 = call-poly "CoreLib.data 2 byte array.vi"("string"=w602) -> ("byteArray out"=w601:T1)  [unwired: 18 in]
            }
          }
          n249 = Unbundle By Name(w593) -> ("code"=w597:i32)
          n250 = Bundle By Name(cluster=w590, "Data"=w584, "Error #"=w597) -> (w596:T2)
        }
        frame "SetLoopMode" {
          n251 = Unbundle By Name(w622) -> ("Data"=w619:T1)
          n252 = call-poly "CoreLib.byte array 2 data.vi"("byteArray"=w619) -> ("i16"=w620:i16, "error out"=w618:errorcluster)  [unwired: 16 in, 1 out]
          n253 = Not Equal To 0?(x=w620) -> (x != 0?=w617:bool)
          n254 = case shown="No Error" w618 {
            tunnel: [w638 w646] -> w627
            tunnel: w631 -> [w642 w646]
            tunnel: w630 -> [w641 w645]
            tunnel: [w636 w644] -> w626
            tunnel: w624 -> [_ w643]
            tunnel: w617 -> [w640 _]
            frame No Error {
              n255 = call "NF87XX.enable closed loop mode.vi"("i ref in"=w642, "Enable closed loop mode"=w640, "error in (no error)"=w641) -> ("i ref out"=w639:refnum<vi>, "error out"=w637:errorcluster)  [unwired: 15 in]
              n256 = call "NF87XX.get status.vi"("i ref in"=w639, "error in (no error)"=w637) -> ("i ref out"=w638:refnum<vi>, "error out"=w636:errorcluster)  [unwired: 15 in, 1 out]
            }
            frame Error {
              n257 = call "CoreLib.set data type mismatch.vi"("error in (no error)"=w645, "error source"=w643) -> ("error out"=w644:errorcluster)  [unwired: 17 in]
            }
          }
          n258 = call "BaseProcess.set event status.vi"("i ref in"=w627, "EventStatus"=w624, "error in (no error)"=w626) -> ("i ref out"=w623:refnum<vi>, "error out"=w625:errorcluster)  [unwired: 14 in, 1 out]
          n259 = case shown="No Error" w625 {
            selector: w625 -> [_ w635]
            tunnel: [T1 [] ("byteArray out") w633] -> w621
            frame No Error {
            }
            frame Error {
              n260 = Unbundle By Name(w635) -> ("source"=w634:string)
              n261 = call-poly "CoreLib.data 2 byte array.vi"("string"=w634) -> ("byteArray out"=w633:T1)  [unwired: 18 in]
            }
          }
          n262 = Unbundle By Name(w625) -> ("code"=w629:i32)
          n263 = Bundle By Name(cluster=w622, "Data"=w621, "Error #"=w629) -> (w628:T2)
        }
        frame "GetPosition" {
          n264 = call "NF87XX.get position.vi"("i ref in"=w652, "error in (no error)"=w651) -> ("i ref out"=w650:refnum<vi>, "error out"=w648:errorcluster)  [unwired: 15 in, 1 out]
          n265 = call "NF87XX.get status.vi"("i ref in"=w650, "error in (no error)"=w648) -> ("i ref out"=w649:refnum<vi>, "error out"=w647:errorcluster)  [unwired: 15 in, 1 out]
          n266 = call "BaseProcess.set event status.vi"("i ref in"=w649, "EventStatus"=w656, "error in (no error)"=w647) -> ("i ref out"=w655:refnum<vi>, "error out"=w657:errorcluster)  [unwired: 14 in, 1 out]
          n267 = Unbundle By Name(w657) -> ("code"=w659:i32)
          n268 = case shown="No Error" w657 {
            selector: w657 -> [_ w663]
            tunnel: [T1 [] ("byteArray out") w661] -> w653
            frame No Error {
            }
            frame Error {
              n269 = Unbundle By Name(w663) -> ("source"=w662:string)
              n270 = call-poly "CoreLib.data 2 byte array.vi"("string"=w662) -> ("byteArray out"=w661:T1)  [unwired: 18 in]
            }
          }
          n271 = Bundle By Name(cluster=w654, "Data"=w653, "Error #"=w659) -> (w658:T2)
        }
        frame "SetPosition" {
          n272 = Unbundle By Name(w668) -> ("Data"=w671:T1)
          n273 = call-poly "CoreLib.byte array 2 data.vi"("byteArray"=w671) -> ("byteArray out"=w670:T1, "string"=w667:string, "error out"=w669:errorcluster)  [unwired: 16 in]
          n274 = call-poly "CoreLib.byte array 2 data.vi"("byteArray"=w670, "error in (no error)"=w669) -> ("i32"=w666:i32, "error out"=w665:errorcluster)  [unwired: 15 in, 1 out]
          n275 = case shown="No Error" w665 {
            tunnel: w675 -> [w688 w692]
            tunnel: w674 -> [w687 w690]
            tunnel: [w683 w690] -> w673
            tunnel: [w681 w691] -> w672
            tunnel: w667 -> [w686 _]
            tunnel: w666 -> [w685 _]
            tunnel: w664 -> [_ w689]
            frame No Error {
              n276 = call "NF87XX.set position.vi"("i ref in"=w687, "System"=w686, "position"=w685, "error in (no error)"=w688) -> ("i ref out"=w684:refnum<vi>, "error out"=w682:errorcluster)  [unwired: 14 in]
              n277 = call "NF87XX.get status.vi"("i ref in"=w684, "error in (no error)"=w682) -> ("i ref out"=w683:refnum<vi>, "error out"=w681:errorcluster)  [unwired: 15 in, 1 out]
            }
            frame Error {
              n278 = call "CoreLib.set data type mismatch.vi"("error in (no error)"=w692, "error source"=w689) -> ("error out"=w691:errorcluster)  [unwired: 17 in]
            }
          }
          n279 = call "BaseProcess.set event status.vi"("i ref in"=w673, "EventStatus"=w664, "error in (no error)"=w672) -> ("i ref out"=w677:refnum<vi>, "error out"=w678:errorcluster)  [unwired: 14 in, 1 out]
          n280 = Unbundle By Name(w678) -> ("code"=w680:i32)
          n281 = case shown="No Error" w678 {
            selector: w678 -> [_ w696]
            tunnel: [T1 [] ("byteArray out") w694] -> w676
            frame No Error {
            }
            frame Error {
              n282 = Unbundle By Name(w696) -> ("source"=w695:string)
              n283 = call-poly "CoreLib.data 2 byte array.vi"("string"=w695) -> ("byteArray out"=w694:T1)  [unwired: 18 in]
            }
          }
          n284 = Bundle By Name(cluster=w668, "Data"=w676, "Error #"=w680) -> (w679:T2)
        }
        frame "SetRelPosition" {
          n285 = Unbundle By Name(w708) -> ("Data"=w700:T1)
          n286 = call-poly "CoreLib.byte array 2 data.vi"("byteArray"=w700) -> ("byteArray out"=w699:T1, "string"=w697:string, "error out"=w698:errorcluster)  [unwired: 16 in]
          n287 = call-poly "CoreLib.byte array 2 data.vi"("byteArray"=w699, "error in (no error)"=w698) -> ("byteArray out"=w701:T1, "i32"=w702:i32, "error out"=w705:errorcluster)  [unwired: 15 in]
          n288 = call-poly "CoreLib.byte array 2 data.vi"("byteArray"=w701, "error in (no error)"=w705) -> ("i16"=w706:i16, "error out"=w704:errorcluster)  [unwired: 15 in, 1 out]
          n289 = Not Equal To 0?(x=w706) -> (x != 0?=w703:bool)
          n290 = case shown="No Error" w704 {
            tunnel: [w724 w734] -> w713
            tunnel: w717 -> [w729 w734]
            tunnel: w716 -> [w730 w733]
            tunnel: [w722 w732] -> w712
            tunnel: w710 -> [_ w731]
            tunnel: w702 -> [w728 _]
            tunnel: w703 -> [w727 _]
            tunnel: w697 -> [w726 _]
            frame No Error {
              n291 = call "NF87XX.set relative position.vi"("i ref in"=w729, "System"=w726, "steps"=w728, "Go immediately?"=w727, "error in (no error)"=w730) -> ("i ref out"=w725:refnum<vi>, "error out"=w723:errorcluster)  [unwired: 13 in]
              n292 = call "NF87XX.get status.vi"("i ref in"=w725, "error in (no error)"=w723) -> ("i ref out"=w724:refnum<vi>, "error out"=w722:errorcluster)  [unwired: 15 in, 1 out]
            }
            frame Error {
              n293 = call "CoreLib.set data type mismatch.vi"("error in (no error)"=w733, "error source"=w731) -> ("error out"=w732:errorcluster)  [unwired: 17 in]
            }
          }
          n294 = call "BaseProcess.set event status.vi"("i ref in"=w713, "EventStatus"=w710, "error in (no error)"=w712) -> ("i ref out"=w709:refnum<vi>, "error out"=w711:errorcluster)  [unwired: 14 in, 1 out]
          n295 = case shown="No Error" w711 {
            selector: w711 -> [_ w721]
            tunnel: [T1 [] ("byteArray out") w719] -> w707
            frame No Error {
            }
            frame Error {
              n296 = Unbundle By Name(w721) -> ("source"=w720:string)
              n297 = call-poly "CoreLib.data 2 byte array.vi"("string"=w720) -> ("byteArray out"=w719:T1)  [unwired: 18 in]
            }
          }
          n298 = Unbundle By Name(w711) -> ("code"=w715:i32)
          n299 = Bundle By Name(cluster=w708, "Data"=w707, "Error #"=w715) -> (w714:T2)
        }
        frame "GetStatus" {
          n300 = call "NF87XX.get status.vi"("i ref in"=w741, "error in (no error)"=w740) -> ("i ref out"=w738:refnum<vi>, "status"=w737:string, "error out"=w739:errorcluster)  [unwired: 15 in]
          n301 = call "BaseProcess.set event status.vi"("i ref in"=w738, "EventStatus"=w743, "error in (no error)"=w739) -> ("i ref out"=w742:refnum<vi>, "error out"=w744:errorcluster)  [unwired: 14 in, 1 out]
          n302 = case shown="No Error" w744 {
            selector: w744 -> [_ w752]
            tunnel: w737 -> [w748 _]
            tunnel: [w749 w750] -> w735
            frame No Error {
              n303 = call-poly "CoreLib.data 2 byte array.vi"("string"=w748) -> ("byteArray out"=w749:T1)  [unwired: 18 in]
            }
            frame Error {
              n304 = Unbundle By Name(w752) -> ("source"=w751:string)
              n305 = call-poly "CoreLib.data 2 byte array.vi"("string"=w751) -> ("byteArray out"=w750:T1)  [unwired: 18 in]
            }
          }
          n306 = Unbundle By Name(w744) -> ("code"=w747:i32)
          n307 = Bundle By Name(cluster=w746, "Data"=w735, "Error #"=w747, "Data Descriptor"="C:N") -> (w745:T2)
        }
        frame "Stop" {
          n308 = Unbundle By Name(w753) -> ("Data"=w760:T1)
          n309 = call-poly "CoreLib.byte array 2 data.vi"("byteArray"=w760) -> ("string"=w759:string, "error out"=w758:errorcluster)  [unwired: 16 in, 1 out]
          n310 = case shown="No Error" w758 {
            tunnel: w756 -> [w773 w776]
            tunnel: [w769 w776] -> w755
            tunnel: w757 -> [w772 w775]
            tunnel: [w767 w774] -> w754
            tunnel: w759 -> [w771 _]
            frame No Error {
              n311 = call "NF87XX.stop.vi"("i ref in"=w773, "System"=w771, "error in (no error)"=w772) -> ("i ref out"=w770:refnum<vi>, "error out"=w768:errorcluster)  [unwired: 15 in]
              n312 = call "NF87XX.get status.vi"("i ref in"=w770, "error in (no error)"=w768) -> ("i ref out"=w769:refnum<vi>, "error out"=w767:errorcluster)  [unwired: 15 in, 1 out]
            }
            frame Error {
              n313 = call "CoreLib.set data type mismatch.vi"("error in (no error)"=w775) -> ("error out"=w774:errorcluster)  [unwired: 18 in]
            }
          }
          n314 = call "BaseProcess.set event status.vi"("i ref in"=w755, "EventStatus"=w763, "error in (no error)"=w754) -> ("i ref out"=w762:refnum<vi>, "error out"=w764:errorcluster)  [unwired: 14 in, 1 out]
          n315 = case shown="Error" w764 {
            selector: w764 -> [_ w780]
            tunnel: [T1 [] ("byteArray out") w778] -> w761
            frame No Error {
            }
            frame Error {
              n316 = Unbundle By Name(w780) -> ("source"=w779:string)
              n317 = call-poly "CoreLib.data 2 byte array.vi"("string"=w779) -> ("byteArray out"=w778:T1)  [unwired: 18 in]
            }
          }
          n318 = Unbundle By Name(w764) -> ("code"=w766:i32)
          n319 = Bundle By Name(cluster=w753, "Data"=w761, "Error #"=w766) -> (w765:T2)
        }
        frame "GetMotorType" {
          n320 = Unbundle By Name(w786) -> ("Data"=w788:T1)
          n321 = call-poly "CoreLib.byte array 2 data.vi"("byteArray"=w788) -> ("byteArray out"=w781:T1, "string"=w787:string, "error out"=w785:errorcluster)  [unwired: 16 in]
          n322 = call-poly "CoreLib.byte array 2 data.vi"("byteArray"=w781, "error in (no error)"=w785) -> ("i32"=w782:i32, "error out"=w784:errorcluster)  [unwired: 15 in, 1 out]
          n323 = case shown="No Error" w784 {
            tunnel: w795 -> [w808 w811]
            tunnel: w794 -> [w807 w813]
            tunnel: [w800 w812] -> w793
            tunnel: [w802 w811] -> w792
            tunnel: [w806 NF87XX.motor_Type."not defined" ("Motor Type")] -> w790
            tunnel: w787 -> [w805 _]
            tunnel: w783 -> [_ w810]
            tunnel: w782 -> [w804 _]
            frame No Error {
              n324 = call "NF87XX.get motor type.vi"("i ref in"=w808, "System"=w805, "Motor (0, 1, 2)"=w804, "error in (no error)"=w807) -> ("i ref out"=w803:refnum<vi>, "Motor Type"=w806:T4, "error out"=w801:errorcluster)  [unwired: 13 in]
              n325 = call "NF87XX.get status.vi"("i ref in"=w803, "error in (no error)"=w801) -> ("i ref out"=w802:refnum<vi>, "error out"=w800:errorcluster)  [unwired: 15 in, 1 out]
            }
            frame Error {
              n326 = call "CoreLib.set data type mismatch.vi"("error in (no error)"=w813, "error source"=w810) -> ("error out"=w812:errorcluster)  [unwired: 17 in]
            }
          }
          n327 = call "BaseProcess.set event status.vi"("i ref in"=w792, "EventStatus"=w783, "error in (no error)"=w793) -> ("i ref out"=w796:refnum<vi>, "error out"=w797:errorcluster)  [unwired: 14 in, 1 out]
          n328 = case shown="No Error" w797 {
            selector: w797 -> [_ w818]
            tunnel: w790 -> [w815 _]
            tunnel: [w814 w816] -> w789
            frame No Error {
              n329 = call-poly "CoreLib.data 2 byte array.vi"("i16"=w815) -> ("byteArray out"=w814:T1)  [unwired: 18 in]
            }
            frame Error {
              n330 = Unbundle By Name(w818) -> ("source"=w817:string)
              n331 = call-poly "CoreLib.data 2 byte array.vi"("string"=w817) -> ("byteArray out"=w816:T1)  [unwired: 18 in]
            }
          }
          n332 = Unbundle By Name(w797) -> ("code"=w799:i32)
          n333 = Bundle By Name(cluster=w786, "Data"=w789, "Error #"=w799, "Data Descriptor"="S:1") -> (w798:T2)
        }
        frame "SetMotorType" {
          n334 = Unbundle By Name(w829) -> ("Data"=w822:T1)
          n335 = call-poly "CoreLib.byte array 2 data.vi"("byteArray"=w822) -> ("byteArray out"=w821:T1, "string"=w819:string, "error out"=w820:errorcluster)  [unwired: 16 in]
          n336 = call-poly "CoreLib.byte array 2 data.vi"("byteArray"=w821, "error in (no error)"=w820) -> ("byteArray out"=w828:T1, "i32"=w826:i32, "error out"=w827:errorcluster)  [unwired: 15 in]
          n337 = call-poly "CoreLib.byte array 2 data.vi"("byteArray"=w828, "error in (no error)"=w827) -> ("i32"=w825:i32, "error out"=w824:errorcluster)  [unwired: 15 in, 1 out]
          n338 = case shown="No Error" w824 {
            tunnel: [w845 w855] -> w834
            tunnel: w838 -> [w851 w855]
            tunnel: w837 -> [w850 w854]
            tunnel: [w843 w853] -> w833
            tunnel: w831 -> [_ w852]
            tunnel: w826 -> [w849 _]
            tunnel: w825 -> [w848 _]
            tunnel: w819 -> [w847 _]
            frame No Error {
              n339 = call "NF87XX.set motor type.vi"("i ref in"=w851, "System"=w847, "Motor Type (0,1)"=w849, "Motor (0,1,2)"=w848, "error in (no error)"=w850) -> ("i ref out"=w846:refnum<vi>, "error out"=w844:errorcluster)  [unwired: 13 in]
              n340 = call "NF87XX.get status.vi"("i ref in"=w846, "error in (no error)"=w844) -> ("i ref out"=w845:refnum<vi>, "error out"=w843:errorcluster)  [unwired: 15 in, 1 out]
            }
            frame Error {
              n341 = call "CoreLib.set data type mismatch.vi"("error in (no error)"=w854, "error source"=w852) -> ("error out"=w853:errorcluster)  [unwired: 17 in]
            }
          }
          n342 = call "BaseProcess.set event status.vi"("i ref in"=w834, "EventStatus"=w831, "error in (no error)"=w833) -> ("i ref out"=w830:refnum<vi>, "error out"=w832:errorcluster)  [unwired: 14 in, 1 out]
          n343 = case shown="Error" w832 {
            selector: w832 -> [_ w842]
            tunnel: [T1 [] ("byteArray out") w840] -> w823
            frame No Error {
            }
            frame Error {
              n344 = Unbundle By Name(w842) -> ("source"=w841:string)
              n345 = call-poly "CoreLib.data 2 byte array.vi"("string"=w841) -> ("byteArray out"=w840:T1)  [unwired: 18 in]
            }
          }
          n346 = Unbundle By Name(w832) -> ("code"=w836:i32)
          n347 = Bundle By Name(cluster=w829, "Data"=w823, "Error #"=w836) -> (w835:T2)
        }
        frame "GetVelocity" {
          n348 = Unbundle By Name(w859) -> ("Data"=w860:T1)
          n349 = call-poly "CoreLib.byte array 2 data.vi"("byteArray"=w860) -> ("string"=w857:string, "error out"=w858:errorcluster)  [unwired: 16 in, 1 out]
          n350 = case shown="No Error" w858 {
            tunnel: w872 -> [w886 w890]
            tunnel: w871 -> [w885 w891]
            tunnel: [w879 w889] -> w870
            tunnel: [w877 w890] -> w869
            tunnel: [w884 w887] -> w867
            tunnel: [w883 w887] -> w866
            tunnel: [w882 w887] -> w863
            tunnel: w857 -> [w881 _]
            tunnel: w856 -> [_ w888]
            frame No Error {
              n351 = call "NF87XX.get velocity.vi"("i ref in"=w886, "System"=w881, "error in (no error)"=w885) -> ("i ref out"=w878:refnum<vi>, "velocity Mot 0 [steps/s]"=w884:dbl, "velocity Mot 1 [steps/s]"=w883:dbl, "velocity Mot 2 [steps/s]"=w882:dbl, "error out"=w880:errorcluster)  [unwired: 12 in]
              n352 = call "NF87XX.get status.vi"("i ref in"=w878, "error in (no error)"=w880) -> ("i ref out"=w877:refnum<vi>, "error out"=w879:errorcluster)  [unwired: 15 in, 1 out]
            }
            frame Error {
              w887 = 99999.0 ("velocity Mot 0 [steps/s]")
              n353 = call "CoreLib.set data type mismatch.vi"("error in (no error)"=w891, "error source"=w888) -> ("error out"=w889:errorcluster)  [unwired: 17 in]
            }
          }
          n354 = call-poly "CoreLib.data 2 byte array.vi"("f64"=w867) -> ("byteArray out"=w865:T1)  [unwired: 18 in]
          n355 = call-poly "CoreLib.data 2 byte array.vi"("byteArray"=w865, "f64"=w866) -> ("byteArray out"=w864:T1)  [unwired: 17 in]
          n356 = call-poly "CoreLib.data 2 byte array.vi"("byteArray"=w864, "f64"=w863) -> ("byteArray out"=w861:T1)  [unwired: 17 in]
          n357 = call "BaseProcess.set event status.vi"("i ref in"=w869, "EventStatus"=w856, "error in (no error)"=w870) -> ("i ref out"=w873:refnum<vi>, "error out"=w874:errorcluster)  [unwired: 14 in, 1 out]
          n358 = Unbundle By Name(w874) -> ("code"=w876:i32)
          n359 = case shown="No Error" w874 {
            selector: w874 -> [_ w895]
            tunnel: [w892 w893] -> w862
            tunnel: w861 -> [w892 _]
            frame No Error {
            }
            frame Error {
              n360 = Unbundle By Name(w895) -> ("source"=w894:string)
              n361 = call-poly "CoreLib.data 2 byte array.vi"("string"=w894) -> ("byteArray out"=w893:T1)  [unwired: 18 in]
            }
          }
          n362 = Bundle By Name(cluster=w859, "Data"=w862, "Error #"=w876, "Data Descriptor"="D:1;D:1;D:1") -> (w875:T2)
        }
        frame "SetVelocity" {
          n363 = Unbundle By Name(w906) -> ("Data"=w899:T1)
          n364 = call-poly "CoreLib.byte array 2 data.vi"("byteArray"=w899) -> ("byteArray out"=w898:T1, "string"=w896:string, "error out"=w897:errorcluster)  [unwired: 16 in]
          n365 = call-poly "CoreLib.byte array 2 data.vi"("byteArray"=w898, "error in (no error)"=w897) -> ("byteArray out"=w905:T1, "d64"=w903:dbl, "error out"=w904:errorcluster)  [unwired: 15 in]
          n366 = call-poly "CoreLib.byte array 2 data.vi"("byteArray"=w905, "error in (no error)"=w904) -> ("i32"=w902:i32, "error out"=w901:errorcluster)  [unwired: 15 in, 1 out]
          n367 = case shown="No Error" w901 {
            tunnel: [w922 w932] -> w911
            tunnel: w915 -> [w928 w932]
            tunnel: w914 -> [w927 w931]
            tunnel: [w920 w930] -> w910
            tunnel: w908 -> [_ w929]
            tunnel: w903 -> [w926 _]
            tunnel: w902 -> [w925 _]
            tunnel: w896 -> [w924 _]
            frame No Error {
              n368 = call "NF87XX.set velocity.vi"("i ref in"=w928, "System"=w924, "velocity (1 .. 2000)"=w926, "Motor (0,1,2)"=w925, "error in (no error)"=w927) -> ("i ref out"=w923:refnum<vi>, "error out"=w921:errorcluster)  [unwired: 13 in]
              n369 = call "NF87XX.get status.vi"("i ref in"=w923, "error in (no error)"=w921) -> ("i ref out"=w922:refnum<vi>, "error out"=w920:errorcluster)  [unwired: 15 in, 1 out]
            }
            frame Error {
              n370 = call "CoreLib.set data type mismatch.vi"("error in (no error)"=w931, "error source"=w929) -> ("error out"=w930:errorcluster)  [unwired: 17 in]
            }
          }
          n371 = call "BaseProcess.set event status.vi"("i ref in"=w911, "EventStatus"=w908, "error in (no error)"=w910) -> ("i ref out"=w907:refnum<vi>, "error out"=w909:errorcluster)  [unwired: 14 in, 1 out]
          n372 = case shown="Error" w909 {
            selector: w909 -> [_ w919]
            tunnel: [T1 [] ("byteArray out") w917] -> w900
            frame No Error {
            }
            frame Error {
              n373 = Unbundle By Name(w919) -> ("source"=w918:string)
              n374 = call-poly "CoreLib.data 2 byte array.vi"("string"=w918) -> ("byteArray out"=w917:T1)  [unwired: 18 in]
            }
          }
          n375 = Unbundle By Name(w909) -> ("code"=w913:i32)
          n376 = Bundle By Name(cluster=w906, "Data"=w900, "Error #"=w913) -> (w912:T2)
        }
        frame "GetMacAddress" {
          n377 = call "NF87XX.get MAC Address.vi"("i ref in"=w942, "error in (no error)"=w941) -> ("i ref out"=w936:refnum<vi>, "MAC Address"=w939:string, "error out"=w934:errorcluster)  [unwired: 15 in]
          n378 = call "NF87XX.get status.vi"("i ref in"=w936, "error in (no error)"=w934) -> ("i ref out"=w935:refnum<vi>, "error out"=w933:errorcluster)  [unwired: 15 in, 1 out]
          n379 = call-poly "CoreLib.data 2 byte array.vi"("string"=w939) -> ("byteArray out"=w938:T1)  [unwired: 18 in]
          n380 = call "BaseProcess.set event status.vi"("i ref in"=w935, "EventStatus"=w944, "error in (no error)"=w933) -> ("i ref out"=w943:refnum<vi>, "error out"=w945:errorcluster)  [unwired: 14 in, 1 out]
          n381 = case shown="No Error" w945 {
            selector: w945 -> [_ w952]
            tunnel: w938 -> [w949 _]
            tunnel: [w949 w950] -> w937
            frame No Error {
            }
            frame Error {
              n382 = Unbundle By Name(w952) -> ("source"=w951:string)
              n383 = call-poly "CoreLib.data 2 byte array.vi"("string"=w951) -> ("byteArray out"=w950:T1)  [unwired: 18 in]
            }
          }
          n384 = Unbundle By Name(w945) -> ("code"=w948:i32)
          n385 = Bundle By Name(cluster=w947, "Data"=w937, "Error #"=w948, "Data Descriptor"="C:N") -> (w946:T2)
        }
        frame "GetHostname" {
          n386 = call "NF87XX.get Hostname.vi"("i ref in"=w962, "error in (no error)"=w961) -> ("i ref out"=w956:refnum<vi>, "Hostname"=w959:string, "error out"=w954:errorcluster)  [unwired: 15 in]
          n387 = call "NF87XX.get status.vi"("i ref in"=w956, "error in (no error)"=w954) -> ("i ref out"=w955:refnum<vi>, "error out"=w953:errorcluster)  [unwired: 15 in, 1 out]
          n388 = call-poly "CoreLib.data 2 byte array.vi"("string"=w959) -> ("byteArray out"=w958:T1)  [unwired: 18 in]
          n389 = call "BaseProcess.set event status.vi"("i ref in"=w955, "EventStatus"=w964, "error in (no error)"=w953) -> ("i ref out"=w963:refnum<vi>, "error out"=w965:errorcluster)  [unwired: 14 in, 1 out]
          n390 = case shown="Error" w965 {
            selector: w965 -> [_ w972]
            tunnel: w958 -> [w969 _]
            tunnel: [w969 w970] -> w957
            frame No Error {
            }
            frame Error {
              n391 = Unbundle By Name(w972) -> ("source"=w971:string)
              n392 = call-poly "CoreLib.data 2 byte array.vi"("string"=w971) -> ("byteArray out"=w970:T1)  [unwired: 18 in]
            }
          }
          n393 = Unbundle By Name(w965) -> ("code"=w968:i32)
          n394 = Bundle By Name(cluster=w967, "Data"=w957, "Error #"=w968, "Data Descriptor"="C:N") -> (w966:T2)
        }
        frame Default {
          n395 = call "BaseProcess.ProcCases.vi"("i ref in"=w975, "selector"=w973, "Data"=w974, "call cluster"=w976, "error in (no error)"=w979) -> ("i ref out"=w980:refnum<vi>, "answer cluster"=w977:T2, "error out"=w978:errorcluster)  [unwired: 12 in]
        }
        frame "RelMove" {
          n396 = Unbundle By Name(w1006) -> ("Data"=w984:T1)
          n397 = call-poly "CoreLib.byte array 2 data.vi"("byteArray"=w984) -> ("byteArray out"=w983:T1, "string"=w981:string, "error out"=w982:errorcluster)  [unwired: 16 in]
          n398 = call-poly "CoreLib.byte array 2 data.vi"("byteArray"=w983, "error in (no error)"=w982) -> ("byteArray out"=w998:T1, "i32"=w985:i32, "error out"=w997:errorcluster)  [unwired: 15 in]
          n399 = call-poly "CoreLib.byte array 2 data.vi"("byteArray"=w998, "error in (no error)"=w997) -> ("byteArray out"=w992:T1, "i32"=w986:i32, "error out"=w991:errorcluster)  [unwired: 15 in]
          n400 = call-poly "CoreLib.byte array 2 data.vi"("byteArray"=w992, "error in (no error)"=w991) -> ("byteArray out"=w996:T1, "d64"=w987:dbl, "error out"=w995:errorcluster)  [unwired: 15 in]
          n401 = call-poly "CoreLib.byte array 2 data.vi"("byteArray"=w996, "error in (no error)"=w995) -> ("byteArray out"=w994:T1, "d64"=w988:dbl, "error out"=w993:errorcluster)  [unwired: 15 in]
          n402 = call-poly "CoreLib.byte array 2 data.vi"("byteArray"=w994, "error in (no error)"=w993) -> ("d64"=w989:dbl, "error out"=w990:errorcluster)  [unwired: 15 in, 1 out]
          n403 = case shown="No Error" w990 {
            tunnel: [w1016 w1029] -> w1004
            tunnel: w1009 -> [w1025 w1029]
            tunnel: w1008 -> [w1024 w1028]
            tunnel: [w1014 w1027] -> w1003
            tunnel: w1001 -> [_ w1026]
            tunnel: w985 -> [w1023 _]
            tunnel: w986 -> [w1022 _]
            tunnel: w987 -> [w1021 _]
            tunnel: w988 -> [w1020 _]
            tunnel: w989 -> [w1019 _]
            tunnel: w981 -> [w1018 _]
            frame No Error {
              n404 = call "NF87XX.relative move.vi"("i ref in"=w1025, "steps (-2147483648 .. 2147483648)"=w1022, "acceleration (16 .. 20000)"=w1021, "start velocity (0 .. 1999)"=w1020, "velocity (1 .. 2000)"=w1019, "error in (no error)"=w1024, "Motor (0, 1 or 2)"=w1023, "System"=w1018) -> ("i ref out"=w1017:refnum<vi>, "error out"=w1015:errorcluster)  [unwired: 10 in]
              n405 = call "NF87XX.get status.vi"("i ref in"=w1017, "error in (no error)"=w1015) -> ("i ref out"=w1016:refnum<vi>, "error out"=w1014:errorcluster)  [unwired: 15 in, 1 out]
            }
            frame Error {
              n406 = call "CoreLib.set data type mismatch.vi"("error in (no error)"=w1028, "error source"=w1026) -> ("error out"=w1027:errorcluster)  [unwired: 17 in]
            }
          }
          n407 = call "BaseProcess.set event status.vi"("i ref in"=w1004, "EventStatus"=w1001, "error in (no error)"=w1003) -> ("i ref out"=w1000:refnum<vi>, "error out"=w1002:errorcluster)  [unwired: 14 in, 1 out]
          n408 = Unbundle By Name(w1002) -> ("code"=w1007:i32)
          n409 = case shown="No Error" w1002 {
            selector: w1002 -> [_ w1013]
            tunnel: [T1 [] ("byteArray out") w1011] -> w999
            frame No Error {
            }
            frame Error {
              n410 = Unbundle By Name(w1013) -> ("source"=w1012:string)
              n411 = call-poly "CoreLib.data 2 byte array.vi"("string"=w1012) -> ("byteArray out"=w1011:T1)  [unwired: 18 in]
            }
          }
          n412 = Bundle By Name(cluster=w1006, "Data"=w999, "Error #"=w1007) -> (w1005:T2)
        }
        frame "AbsMove" {
          n413 = Unbundle By Name(w1047) -> ("Data"=w1037:T1)
          n414 = call-poly "CoreLib.byte array 2 data.vi"("byteArray"=w1037) -> ("byteArray out"=w1034:T1, "string"=w1033:string, "error out"=w1035:errorcluster)  [unwired: 16 in]
          n415 = call-poly "CoreLib.byte array 2 data.vi"("byteArray"=w1034, "error in (no error)"=w1035) -> ("byteArray out"=w1039:T1, "i16"=w1031:i16, "error out"=w1038:errorcluster)  [unwired: 15 in]
          n416 = Greater Than 0?(x=w1031) -> (x > 0?=w1030:bool)
          n417 = call-poly "CoreLib.byte array 2 data.vi"("byteArray"=w1039, "error in (no error)"=w1038) -> ("d64"=w1032:dbl, "error out"=w1036:errorcluster)  [unwired: 15 in, 1 out]
          n418 = case shown="No Error" w1036 {
            tunnel: [w1060 w1067] -> w1045
            tunnel: w1050 -> [w1063 w1067]
            tunnel: w1049 -> [w1062 w1066]
            tunnel: [w1058 w1065] -> w1044
            tunnel: w1042 -> [_ w1064]
            tunnel: w1030 -> [w1056 _]
            tunnel: w1033 -> [w1057 _]
            tunnel: w1032 -> [w1055 _]
            frame No Error {
              n419 = call "NF87XX.absolute move.vi"("i ref in"=w1063, "System"=w1057, "forward?"=w1056, "velocity (1 .. 2000)"=w1055, "error in (no error)"=w1062) -> ("i ref out"=w1061:refnum<vi>, "error out"=w1059:errorcluster)  [unwired: 13 in]
              n420 = call "NF87XX.get status.vi"("i ref in"=w1061, "error in (no error)"=w1059) -> ("i ref out"=w1060:refnum<vi>, "error out"=w1058:errorcluster)  [unwired: 15 in, 1 out]
            }
            frame Error {
              n421 = call "CoreLib.set data type mismatch.vi"("error in (no error)"=w1066, "error source"=w1064) -> ("error out"=w1065:errorcluster)  [unwired: 17 in]
            }
          }
          n422 = call "BaseProcess.set event status.vi"("i ref in"=w1045, "EventStatus"=w1042, "error in (no error)"=w1044) -> ("i ref out"=w1041:refnum<vi>, "error out"=w1043:errorcluster)  [unwired: 14 in, 1 out]
          n423 = Unbundle By Name(w1043) -> ("code"=w1048:i32)
          n424 = case shown="No Error" w1043 {
            selector: w1043 -> [_ w1054]
            tunnel: [T1 [] ("byteArray out") w1052] -> w1040
            frame No Error {
            }
            frame Error {
              n425 = Unbundle By Name(w1054) -> ("source"=w1053:string)
              n426 = call-poly "CoreLib.data 2 byte array.vi"("string"=w1053) -> ("byteArray out"=w1052:T1)  [unwired: 18 in]
            }
          }
          n427 = Bundle By Name(cluster=w1047, "Data"=w1040, "Error #"=w1048) -> (w1046:T2)
        }
        frame "Reset" {
          n428 = call "NF87XX.reset.vi"("i ref in"=w1074, "error in (no error)"=w1073) -> ("i ref out"=w1071:refnum<vi>, "error out"=w1070:errorcluster)  [unwired: 16 in]
          n429 = call "NF87XX.get status.vi"("i ref in"=w1071, "error in (no error)"=w1070) -> ("i ref out"=w1068:refnum<vi>, "error out"=w1069:errorcluster)  [unwired: 15 in, 1 out]
          n430 = call "BaseProcess.set event status.vi"("i ref in"=w1068, "EventStatus"=w1076, "error in (no error)"=w1069) -> ("i ref out"=w1075:refnum<vi>, "error out"=w1077:errorcluster)  [unwired: 14 in, 1 out]
          n431 = case shown="Error" w1077 {
            selector: w1077 -> [_ w1084]
            tunnel: [T1 [] ("byteArray out") w1082] -> w1072
            frame No Error {
            }
            frame Error {
              n432 = Unbundle By Name(w1084) -> ("source"=w1083:string)
              n433 = call-poly "CoreLib.data 2 byte array.vi"("string"=w1083) -> ("byteArray out"=w1082:T1)  [unwired: 18 in]
            }
          }
          n434 = Unbundle By Name(w1077) -> ("code"=w1080:i32)
          n435 = Bundle By Name(cluster=w1079, "Data"=w1072, "Error #"=w1080) -> (w1078:T2)
        }
      }
    }
    frame Error {
    }
  }
  "answer cluster" <- w7
  "i ref out" <- w4
  "error out" <- w3
